vi "Host_1_00.vi"() -> ()   [LabVIEW 2015]
uses:
  <vilib>/userdefined/High Color/nirio_resource_hc.ctl
  <vilib>/FPGAPlugInAG/PCIe-1473R-LX110/niLvFpga_Open_PCIe-1473R-LX110.vi
  <vilib>/rvi/interface/common/dynamic/niFpgaDynamicAddResources.vi
  <vilib>/FPGAPlugInAG/Dynamic/niLvFpga_Reset_Dynamic.vi
  <vilib>/Utility/error.llb/Error Cluster From Error Code.vi
  <vilib>/rvi/errors/niLvFpgaAdjustHostInterfaceError.vi
  <vilib>/FPGAPlugInAG/Dynamic/niLvFpga_Run_Dynamic.vi
  <vilib>/rvi/interface/common/niFpgaWaitOnOcc.vi
  <vilib>/FPGAPlugInAG/Dynamic/niLvFpga_Close_Dynamic.vi
  <vilib>/rvi/interface/nirviOpenFPGA/nirviOpenFPGA.xnode
  1-Tap8-BitCamera_FPGATarget2_FPGA8tapNI_o7jHY7Rbrto.lvbitx
  <vilib>/rvi/interface/nirviMethod/nirviMethod.xnode
  <vilib>/rvi/interface/nirviReadWriteControl/nirviReadWriteControl.xnode
  <vilib>/rvi/interface/nirviCloseFPGA/nirviCloseFPGA.xnode
  NiFpgaLv.dll
  <vilib>/rvi/interface/Simulation/niFpgaSimulationCallBeginRW.vi
  <vilib>/FPGAPlugInAG/Dynamic/niLvFpga_ReadFifo_Dynamic.vi
  <vilib>/rvi/errors/niLvFpgaMergeErrorWithErrorCode.vi
  <vilib>/FPGAPlugInAG/Dynamic/niLvFpga_ConfigureFifo_Dynamic.vi
  <vilib>/FPGAPlugInAG/Dynamic/niLvFpga_StartFifo_Dynamic.vi
panel:
  in  "RIO Device":T1="RIO0"
  in  "Start Serial Server":bool=TRUE
  out "Acq'd Frame Height":u32
  out "Frames Acq'd":u32
  out "DMA Write Timeout":bool
  out "Acq'd Frame Width":u32
  in  "Stopped":bool
  out "Acq In Progress":bool
  in  "Bayer Pattern":u16(ring) items=["GBGB::RGRG", "GRGR::BGBG", "BGBG::GRGR", "RGRG::GBGB"]
  out "Image Width 2":u32=2048 max=65535
  out "Image":T2(plugin-control)
  in  "Acquire":bool
  in  "Frames To Acquire":u32=1 caption="Frames To Acquire\n(0 = infinite)"
  in  "Stop":bool
  in  "Cancel":bool
  in  "Image Height":u32=2048 max=65535
  in  "Image Width":u32=2048 max=65535
  out "Initialized":bool
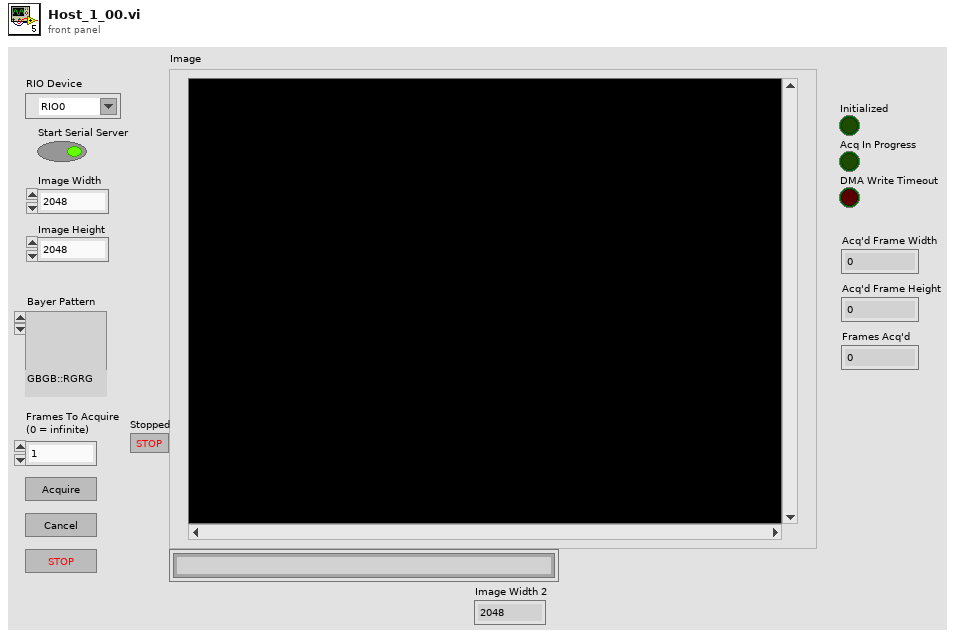
[diagram p1: front panel]
types:
  T1 = typedef "nirio_resource_hc.ctl" = tag
  T2 = typedef "IMAQ Image.ctl" = refnum<image>
  T3 = enum8{"Standard", "Basler 10-tap", "Vosskühler 10-tap"}
  T4 = typedef "Image Type" = u32
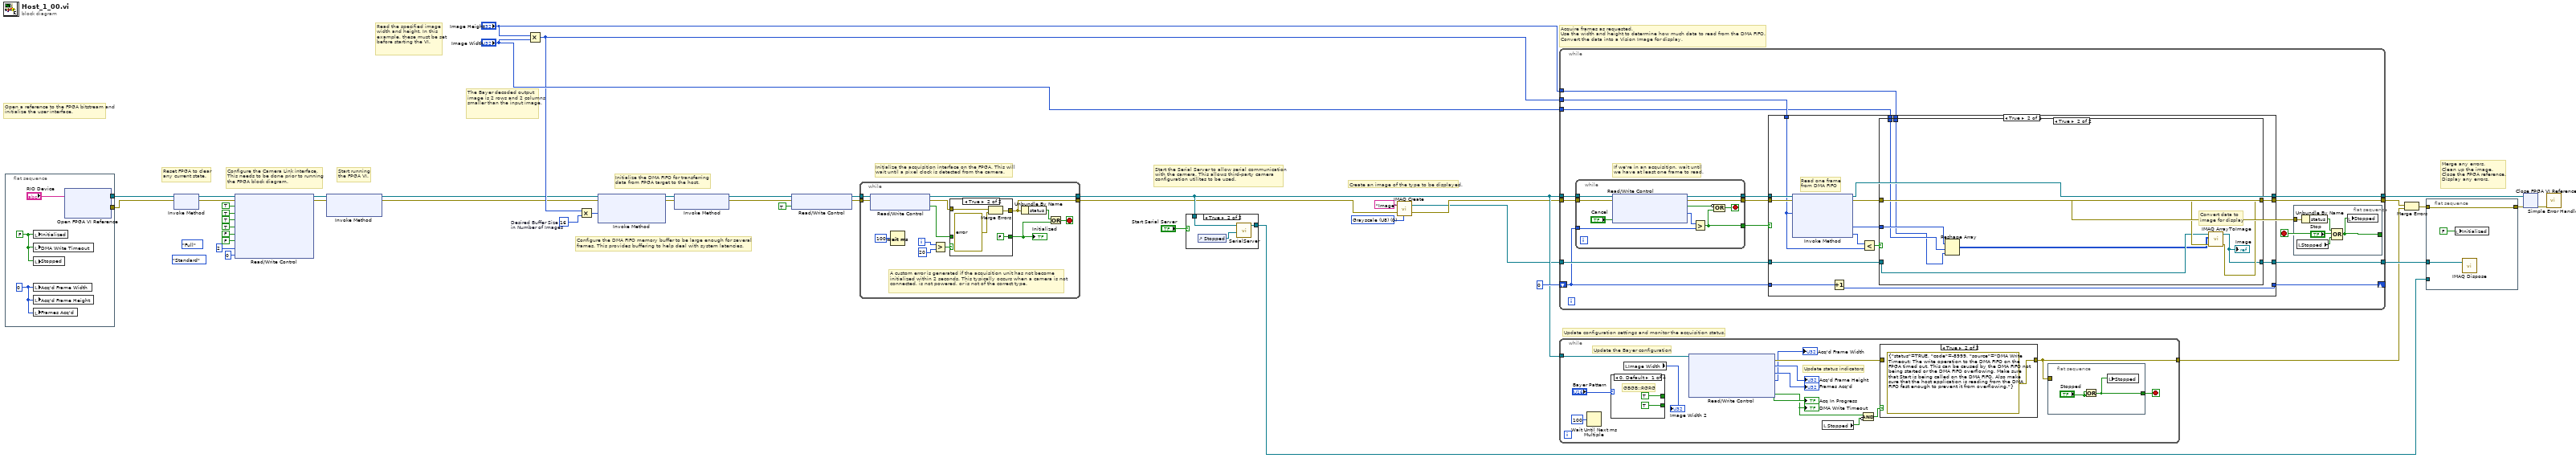
[diagram p0: block diagram]
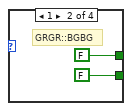
[diagram p3: hidden frame]
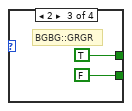
[diagram p4: hidden frame]
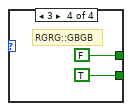
[diagram p5: hidden frame]
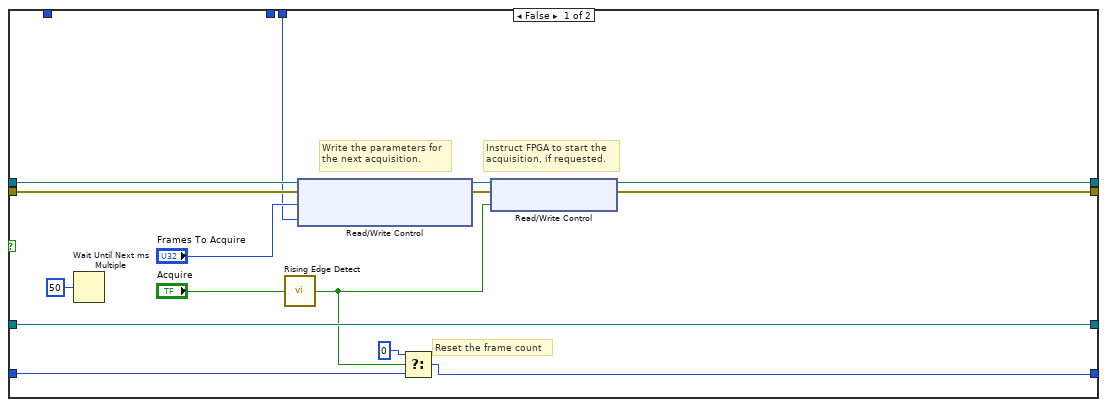
[diagram p7: hidden frame]
diagram:
  (unwired) enum8{"Base", "Medium", "Full"}."Full" ("CL Config.Configuration")
  (unwired) T3."Standard" ("CL Config.Signal Mapping")
  w40 = T4 0 items=["Grayscale (U8)", "Grayscale (I16)", "Grayscale (SGL)", "Complex (CSG)", "RGB (U32)", "HSL (U32)", "RGB (U64)", "Grayscale (U16)"] ("Image Type")
  w14 = u32 16  # Desired Buffer Size in Number of Images
  # "The Bayer decoded output image is 2 rows and 2 columns smaller than the input image."
  # "Configure the DMA FIFO memory buffer to be large enough for several\nframes. This provides buffering to help deal with system latencies."
  # "Start running\nthe FPGA VI."
  # "Reset FPGA to clear\nany current state."
  # "Read the specified image width and height. In this example, these must be set before starting the VI."
  # "Merge any errors.\nClean up the image.\nClose the FPGA reference.\nDisplay any errors."
  # "Acquire frames as requested.\nUse the width and height to determine how much data to read from the DMA FIFO.\nConvert the data into a Vision Image for display."
  # "Update configuration settings and monitor the acquisition status."
  # "Start the Serial Server to allow serial communication\nwith the camera. This allows third-party camera\nconfiguration utilites to be used."
  # "Create an image of the type to be displayed."
  # "Initialize the acquisition interface on the FPGA. This will\nwait until a pixel clock is detected from the camera."
  # "Initialize the DMA FIFO for transferring\ndata from FPGA target to the host."
  # "Configure the Camera Link interface.\nThis needs to be done prior to running\nthe FPGA block diagram."
  # "Open a reference to the FPGA bitstream and initialize the user interface."
  n1 = flat-sequence {
    tunnel: [w46] -> w33
    tunnel: [w45] -> w44
    frame #0 {
      w49 = u32 0 ("Num Lines Acq'd")
      w48 = FALSE ("stop")
      n2 = local write "Initialized"(w48) -> ()
      n3 = local write "DMA Write Timeout"(w48) -> ()
      n4 = local write "Stopped"(w48) -> ()
      n5 = local write "Acq'd Frame Width"(w49) -> ()
      n6 = local write "Acq'd Frame Height"(w49) -> ()
      n7 = local write "Frames Acq'd"(w49) -> ()
      n8 = xnode "Open FPGA VI Reference"("resource name"="RIO Device") -> ("FPGA VI Reference Out"=w46:refnum<k20>, "error out"=w45:errorcluster)  [unwired: 1 in]
    }
  }
  n9 = xnode "Invoke Method"("FPGA VI Reference In"=w33, "error in"=w44) -> ("FPGA VI Reference Out"=w22:refnum<k20>, "error out"=w25:errorcluster)
  n10 = xnode "Read/Write Control"("FPGA VI Reference In"=w22, "error in"=w25, "CL Config.FVAL Active High"=TRUE ("IO Module Config.CL FVAL Active High"), "CL Config.LVAL Active High"=TRUE ("IO Module Config.CL LVAL Active High"), "CL Config.DVAL Active High"=TRUE ("IO Module Config.CL DVAL Active High"), "CL Config.Spare Active High"=TRUE ("IO Module Config.CL Spare Active High"), "CL Config.Line Scan"=FALSE ("Line Scan"), "Acq Control.Ignore DVAL"=FALSE ("CL Config.Line Scan"), "CL Set Configuration"=u8 2, "CL Set Signal Mapping"=u8 0) -> ("FPGA VI Reference Out"=w26:refnum<k20>, "error out"=w24:errorcluster)
  n11 = xnode "Invoke Method"("FPGA VI Reference In"=w26, "error in"=w24) -> ("FPGA VI Reference Out"=w4:refnum<k20>, "error out"=w3:errorcluster)  [unwired: 1 in]
  n12 = Multiply(x="Image Height", y="Image Width") -> (x*y=w5:u32)
  n13 = Multiply(x=w5, y=w14) -> (x*y=w16:u32)
  n14 = xnode "Invoke Method"("FPGA VI Reference In"=w4, "error in"=w3, "Requested Depth"=w16) -> ("FPGA VI Reference Out"=w32:refnum<k20>, "error out"=w31:errorcluster)  [unwired: 1 out]
  n15 = xnode "Invoke Method"("FPGA VI Reference In"=w32, "error in"=w31) -> ("FPGA VI Reference Out"=w17:refnum<k20>, "error out"=w30:errorcluster)
  n16 = xnode "Read/Write Control"("FPGA VI Reference In"=w17, "error in"=w30, "Acq Control.Initialize"=TRUE ("Arm Acquisition")) -> ("FPGA VI Reference Out"=w43:refnum<k20>, "error out"=w42:errorcluster)
  n17 = while {
    tunnel: w43 -> [w57]
    tunnel: w42 -> [w56]
    tunnel: [w55] -> w13
    tunnel: [w59] -> w12
    i -> [w51]
    stop <- w62 stop-if-true
    # "A custom error is generated if the acquisition unit has not become initialized within 2 seconds. This typically occurs when a camera is not connected, is not powered, or is not of the correct type."
    n18 = xnode "Read/Write Control"("FPGA VI Reference In"=w57, "error in"=w56) -> ("FPGA VI Reference Out"=w55:refnum<k20>, "error out"=w54:errorcluster, "Acq Status.Initialized"=w53:bool)
    n19 = Wait (ms)(milliseconds to wait=u32 100) -> ()  [unwired: 1 out]
    n20 = Greater?(x=w51, y=20) -> (0:w52:bool)
    n21 = case shown="True" w52 {
      tunnel: [w64 FALSE] -> w58
      tunnel: w53 -> [w64 _]
      tunnel: w54 -> [w63 w66]
      tunnel: [w63 w68] -> w59
      frame False {
      }
      frame True {
        n22 = Merge Errors(w66, errorcluster {"status"=TRUE, "code"=-8999, "source"="Acquisition Initialization: This error typically occurs when a camera is not properly connected, is not powered, or is not of the correct type."} ("error in")) -> (w68:errorcluster)
      }
    }
    "Initialized" <- w58
    n23 = Unbundle By Name(w59) -> ("status"=w61:bool)
    n24 = Or(x=w61, y=w58) -> (x .or. y?=w62:bool)
  }
  n25 = case shown="True" "Start Serial Server" {
    tunnel: [_ w69] -> w34
    tunnel: w13 -> [_ w70]
    frame False {
    }
    frame True {
      n26 = control-ref of="Stopped"() -> (w71:refnum<vi>)
      n27 = call "SerialServer.vi"("Stop Refnum"=w71, "FPGA VI Reference In"=w70) -> ("FPGA VI Reference Out"=w69:refnum<k20>)  [unwired: 5 in]
    }
  }
  n28 = call "IMAQ Create"("Image Name"="Image", "Image Type"=w40, "error in (no error)"=w12) -> ("New Image"=w8:T2, "error out"=w9:errorcluster)  [unwired: 2 in]
  n29 = while {
    tunnel: w13 -> [w78]
    tunnel: w9 -> [w77]
    tunnel: w5 -> [w86]
    tunnel: "Image Height" -> [w85]
    tunnel: "Image Width" -> [w84]
    tunnel: w8 -> [w83]
    tunnel: [w81] -> w28
    tunnel: [w82] -> w39
    tunnel: [w79] -> w36
    shift-right: [w73] -> _
    shift-left: u32 0 -> [w72]
    stop <- w80 stop-if-true
    # "If we're in an acquisition, wait until \nwe have at least one frame to read."
    n30 = while {
      tunnel: w78 -> [w93]
      tunnel: w77 -> [w92]
      tunnel: [w90] -> w76
      tunnel: [w91] -> w75
      tunnel: w72 -> [w96]
      tunnel: [w94] -> w74
      stop <- w95 stop-if-true
      n31 = xnode "Read/Write Control"("FPGA VI Reference In"=w93, "error in"=w92, "Acq Control.Cancel Acq"="Cancel") -> ("FPGA VI Reference Out"=w91:refnum<k20>, "error out"=w90:errorcluster, "Acq Status.Acq In Progress"=w89:bool, "Acq Status.Frames Acq'd"=w88:u32)
      n32 = Greater?(x=w88, y=w96) -> (0:w94:bool)
      n33 = Compound Arithmetic op=OR(invert w89, w94) -> (w95:bool)
    }
    n34 = case shown="True" w74 {
      tunnel: w75 -> [w112 w127]
      tunnel: w76 -> [w111 w126]
      tunnel: w86 -> [_ w119]
      tunnel: w85 -> [w109 w121]
      tunnel: w84 -> [_ w122]
      tunnel: w83 -> [w116 w131]
      tunnel: [w105 w129] -> w81
      tunnel: [w108 w117] -> w82
      tunnel: [w116 w128] -> w79
      tunnel: w72 -> [w113 w125]
      tunnel: [w115 w124] -> w73
      frame False {
        # "Reset the frame count"
        # "Instruct FPGA to start the\nacquisition, if requested."
        # "Write the parameters for\nthe next acquisition."
        n35 = Wait Until Next ms Multiple(millisecond multiple=u32 50) -> ()  [unwired: 1 out]
        n36 = call "Rising Edge Detect.vi"("Input"="Acquire") -> ("Pulse"=w102:bool)  [unwired: 4 in]
        n37 = xnode "Read/Write Control"("FPGA VI Reference In"=w112, "error in"=w111, "Acq Control.Frames To Acq"="Frames To Acquire", "Acq Control.Line Scan Height"=w109) -> ("FPGA VI Reference Out"=w107:refnum<k20>, "error out"=w106:errorcluster)
        n38 = Select(t=u32 0, s=w102, f=w113) -> (s? t:f=w115:u32)
        n39 = xnode "Read/Write Control"("FPGA VI Reference In"=w107, "error in"=w106, "Acq Control.Acquire"=w102) -> ("FPGA VI Reference Out"=w108:refnum<k20>, "error out"=w105:errorcluster)
      }
      frame True {
        # "Read one frame\nfrom DMA FIFO"
        n40 = xnode "Invoke Method"("FPGA VI Reference In"=w127, "error in"=w126, "Number of Elements"=w119) -> ("FPGA VI Reference Out"=w117:refnum<k20>, "error out"=w130:errorcluster, "Data"=w123:u8[], "Elements Remaining"=w120:u32)  [unwired: 1 in]
        n41 = Increment(x=w125) -> (x+1=w124:u32)
        n42 = Less?(x=w120, y=w119) -> (x < y?=w118:bool)
        n43 = case shown="True" w118 {
          tunnel: w131 -> [w133 w138]
          tunnel: w130 -> [w132 w139]
          tunnel: [w132 w141] -> w129
          tunnel: [w133 w140] -> w128
          tunnel: w123 -> [_ w137]
          tunnel: w122 -> [_ w136]
          tunnel: w121 -> [_ w135]
          frame False {
            # "Do not display the image if we're\nfalling behind in the acquisition."
          }
          frame True {
            # "Convert data to\nimage for display"
            n44 = Reshape Array(w137, w136, w135) -> (w134:u8[][])
            n45 = call "IMAQ ArrayToImage"("error in (no error)"=w139, "Image Pixels (U8)"=w134, "Image"=w138) -> ("error out"=w141:errorcluster, "Image Out"=w140:T2)  [unwired: 7 in]
            "Image" <- w140
          }
        }
      }
    }
    n46 = flat-sequence {
      tunnel: w81 -> [w99]
      tunnel: [w98] -> w80
      frame #0 {
        n47 = local read "Stopped"() -> (w97:bool)
        n48 = Unbundle By Name(w99) -> ("status"=w100:bool)
        n49 = Compound Arithmetic op=OR(w100, "Stop", w97) -> (w98:bool)
        n50 = local write "Stopped"(w98) -> ()
      }
    }
  }
  n51 = while {
    tunnel: w13 -> [w152]
    tunnel: [w155] -> w27
    stop <- w154 stop-if-true
    # "Update the Bayer configuration"
    # "Update status indicators"
    n52 = Wait Until Next ms Multiple(millisecond multiple=u32 100) -> ()  [unwired: 1 out]
    n53 = case shown="0, Default" "Bayer Pattern" {
      tunnel: [TRUE FALSE TRUE FALSE] -> _
      tunnel: [TRUE FALSE FALSE TRUE] -> _
      frame 0, Default {
        # "GBGB::RGRG"
      }
      frame 1 {
        # "GRGR::BGBG"
      }
      frame 2 {
        # "BGBG::GRGR"
      }
      frame 3 {
        # "RGRG::GBGB"
      }
    }
    n54 = local read "Image Width"() -> (→"Image Width 2":u32)
    n55 = xnode "Read/Write Control"("FPGA VI Reference In"=w152) -> ("error out"=w151:errorcluster, "Acq Status.Lines Per Frame"=→"Acq'd Frame Height":u32, "Acq Status.Frames Acq'd"=→"Frames Acq'd":u32, "Acq Status.Clocks Per Line"=→"Acq'd Frame Width":u32, "Acq Status.Acq In Progress"=→"Acq In Progress":bool, "Acq Status.DMA Write Timeout"=w143:bool)  [unwired: 1 in, 1 out]
    "DMA Write Timeout" <- w143
    n56 = local read "Stopped"() -> (w144:bool)
    n57 = Compound Arithmetic op=AND(w143, invert w144) -> (w145:bool)
    n58 = case shown="True" w145 {
      tunnel: w151 -> [w166 _]
      tunnel: [w166 errorcluster {"status"=TRUE, "code"=-8999, "source"="DMA Write Timeout: The write operation to the DMA FIFO on the FPGA timed out. This can be caused by the DMA FIFO not being started or the DMA FIFO overflowing. Make sure that Start is being called on the DMA FIFO. Also make sure that the host application is reading from the DMA FIFO fast enough to prevent it from overflowing."} ("error out")] -> w155
      frame False {
      }
      frame True {
      }
    }
    n59 = flat-sequence {
      tunnel: w155 -> [_]
      tunnel: [w165] -> w154
      frame #0 {
        n60 = Or(x="Stopped", y="Stopped") -> (x .or. y?=w165:bool)
        n61 = local write "Stopped"(w165) -> ()
      }
    }
  }
  n62 = Merge Errors(w28, w27) -> (w29:errorcluster)
  n63 = flat-sequence {
    tunnel: w29 -> [w169]
    tunnel: [w169] -> w38
    tunnel: w36 -> [w170]
    tunnel: w34 -> [_]
    frame #0 {
      n64 = local write "Initialized"(FALSE ("Module Enabled")) -> ()
      n65 = call "IMAQ Dispose"("Image"=w170) -> ()  [unwired: 5 in, 1 out]
    }
  }
  n66 = xnode "Close FPGA VI Reference"("FPGA VI Reference In"=w39, "error in"=w38) -> ("error out"=w35:errorcluster)
  n67 = call <vilib>:"Simple Error Handler.vi"("error in (no error)"=w35) -> ()  [unwired: 4 in, 5 out]
